vi "Get Ethernet Configuration.vi"(8 "error in (no error)":errorcluster, 11 "Ethernet in":refnum<class "ENET_BS1200.lvclass">) -> (0 "error out":errorcluster, 1 "Configuration Error?":bool, 2 "Ethernet Settings":T1, 3 "Ethernet out":refnum<class "ENET_BS1200.lvclass">)   [LabVIEW 2021, in "BS120x Driver.lvlib" / "ENET_BS1200.lvclass"]
doc: "Retrieve Battery Simulator 1200 Ethernet settings.\n(c) 2019 Bloomy Controls, Inc. All rights reserved."
uses:
  ENET_BS1200.lvclass
  TypeDefs/Ethernet Settings.ctl
  <vilib>/nisyscfg/Close (System).vi
  <vilib>/WebDAVClient/Advanced/Get Buffer.vi
  ENET_BS1200.lvclass/ENET_BS1200.ctl
  <vilib>/WebDAVClient/NI_WebDAV.lvlib
  <resource>/objmgr/nisysapi.rc
  <vilib>/nisyscfg/nisyscfg.lvlib
  BS120x.lvclass
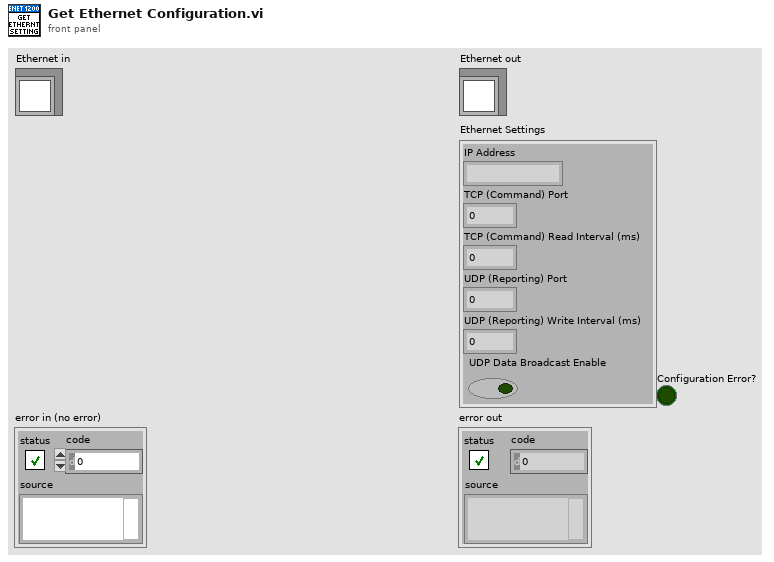
[diagram p1: front panel]
types:
  T1 = typedef "BS120x Driver.lvlib/BS120x.lvclass/Ethernet Settings.ctl" = cluster{"IP Address":string, "TCP (Command) Port":u16, "TCP (Command) Read Interval (ms)":u32, "UDP (Reporting) Port":u16, "UDP (Reporting) Write Interval (ms)":u32, "UDP Data Broadcast Enable":bool}
  T2 = typedef "NI_WebDAV.lvlib/SessionHandle.ctl" = refnum<k1>
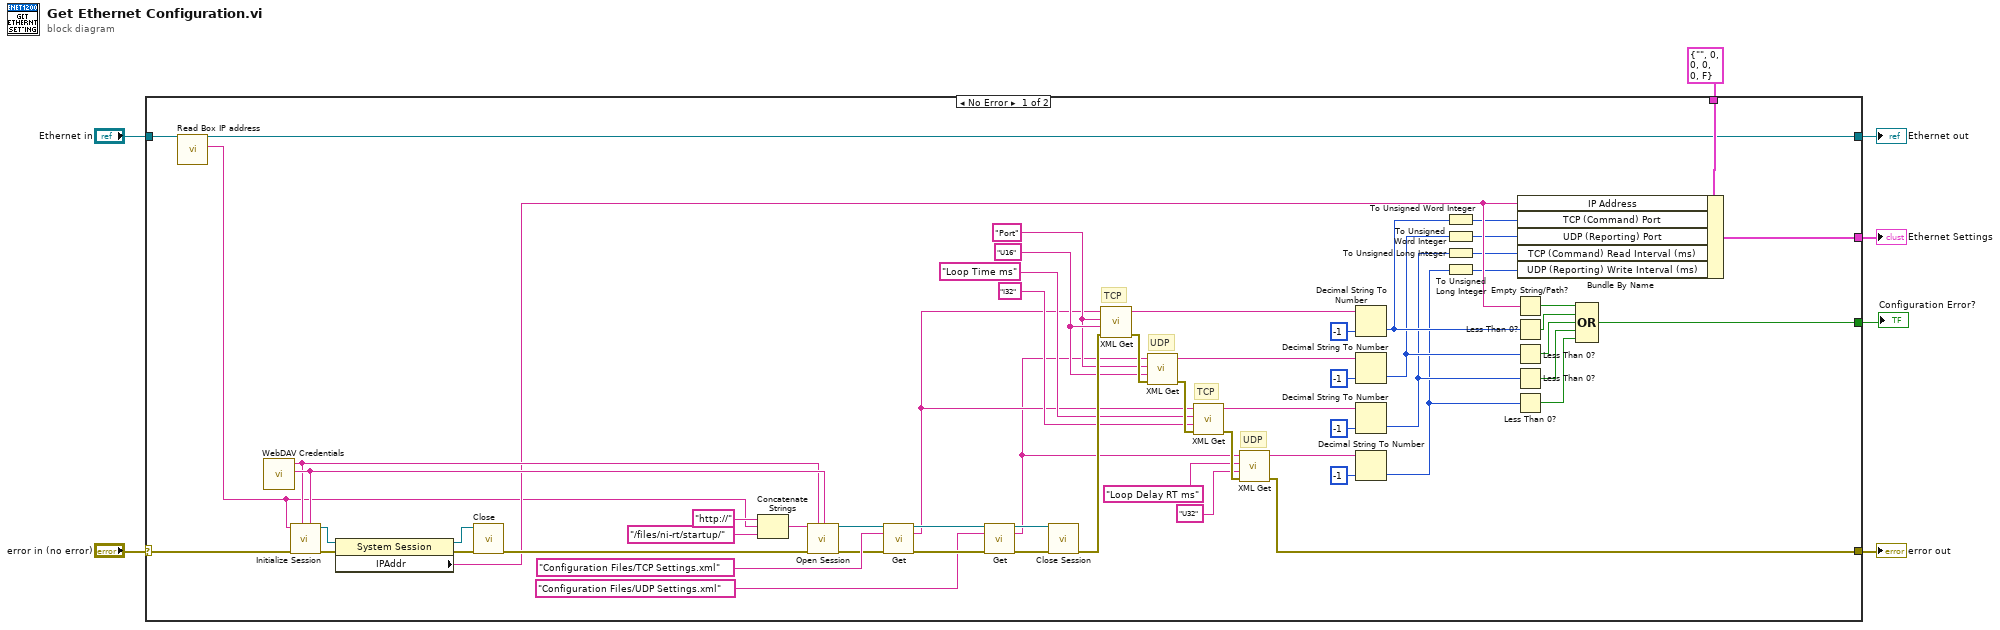
[diagram p0: block diagram]
diagram:
  n1 = case shown="No Error" "error in (no error)" {
    selector: "error in (no error)" -> [w41 w70]
    tunnel: [w46 w70] -> w6
    tunnel: [w9 w69] -> w4
    tunnel: "Ethernet in" -> [w10 w69]
    tunnel: [w66 w68] -> w2
    tunnel: T1 {"IP Address"="", "TCP (Command) Port"=0, "TCP (Command) Read Interval (ms)"=0, "UDP (Reporting) Port"=0, "UDP (Reporting) Write Interval (ms)"=0, "UDP Data Broadcast Enable"=FALSE} ("Ethernet Settings") -> [w67 w68]
    tunnel: [w17 _] -> w1
    frame No Error {
      w43 = "U16" ("Data Type")
      w42 = "Port" ("Parameter")
      # "TCP"
      # "UDP"
      # "UDP"
      # "TCP"
      n2 = call-dynamic "Read Box IP address.vi"("ENET_BS120x in"=w10) -> ("Box IP address"=w8:string, "ENET_BS120x out"=w9:refnum<class "ENET_BS1200.lvclass">)  [unwired: 8 in, 1 out]
      n3 = call "WebDAV Credentials.vi"() -> ("Password"=w35:string, "Username"=w34:string)  [unwired: 10 in]
      n4 = call <vilib>:"Initialize Session.vi"("Password"=w35, "User Name"=w34, "error in (no error)"=w41, "Target (localhost)"=w8) -> ("error out"=w39:errorcluster, "Session out"=w40:refnum<k21>)  [unwired: 6 in]
      n5 = property class="System Session"(reference=w40, error in=w39) -> (reference out=w37:refnum<k21>, error out=w38:errorcluster, "IPAddr"=w27:string)
      n6 = call-poly <vilib>:"Close.vi"("error in (no error)"=w38, "Session in"=w37) -> ("error out"=w36:errorcluster)  [unwired: 9 in]
      n7 = Concatenate Strings("http://" ("string"), w8, "/files/ni-rt/startup/" ("string")) -> (w63:string)
      n8 = call <vilib>:"Open Session.vi"("host uri prefix"=w63, "username"=w34, "password"=w35, "error in (no error)"=w36) -> ("session handle out"=w61:T2, "error out"=w60:errorcluster)  [unwired: 10 in]
      n9 = call-poly <vilib>:"Get.vi"("session handle"=w61, "relative uri"="Configuration Files/TCP Settings.xml" ("string"), "error in (no error)"=w60) -> ("session handle out"=w59:T2, "data"=w12:string, "error out"=w58:errorcluster)  [unwired: 10 in]
      n10 = call-poly <vilib>:"Get.vi"("session handle"=w59, "relative uri"="Configuration Files/UDP Settings.xml" ("string"), "error in (no error)"=w58) -> ("session handle out"=w57:T2, "data"=w11:string, "error out"=w56:errorcluster)  [unwired: 10 in]
      n11 = call <vilib>:"Close Session.vi"("session handle"=w57, "error in (no error)"=w56) -> ("error out"=w53:errorcluster)  [unwired: 13 in]
      n12 = call "XML Get.vi"("error in (no error)"=w53, "Data Type"=w43, "Parameter"=w42, "XML String in"=w12) -> ("error out"=w49:errorcluster, "Value"=w54:string)  [unwired: 6 in]
      n13 = call "XML Get.vi"("error in (no error)"=w49, "Data Type"=w43, "Parameter"=w42, "XML String in"=w11) -> ("error out"=w48:errorcluster, "Value"=w52:string)  [unwired: 6 in]
      n14 = call "XML Get.vi"("error in (no error)"=w48, "Data Type"="I32", "Parameter"="Loop Time ms", "XML String in"=w12) -> ("error out"=w47:errorcluster, "Value"=w51:string)  [unwired: 6 in]
      n15 = call "XML Get.vi"("error in (no error)"=w47, "Data Type"="U32", "Parameter"="Loop Delay RT ms", "XML String in"=w11) -> ("error out"=w46:errorcluster, "Value"=w50:string)  [unwired: 6 in]
      n16 = Decimal String To Number(string=w54, default (0L)=-1 ("default (0 I32)")) -> (number=w26:i32)  [unwired: 1 in, 1 out]
      n17 = Decimal String To Number(string=w52, default (0L)=-1 ("default (0 I32)")) -> (number=w25:i32)  [unwired: 1 in, 1 out]
      n18 = Decimal String To Number(string=w51, default (0L)=-1 ("default (0 I32)")) -> (number=w24:i32)  [unwired: 1 in, 1 out]
      n19 = Decimal String To Number(string=w50, default (0L)=-1 ("default (0 I32)")) -> (number=w23:i32)  [unwired: 1 in, 1 out]
      n20 = To Unsigned Word Integer(number=w26) -> (unsigned 16bit integer=w16:u16)
      n21 = To Unsigned Word Integer(number=w25) -> (unsigned 16bit integer=w15:u16)
      n22 = To Unsigned Long Integer(number=w24) -> (unsigned 32bit integer=w14:u32)
      n23 = To Unsigned Long Integer(number=w23) -> (unsigned 32bit integer=w13:u32)
      n24 = Empty String/Path?(string/path=w27) -> (empty?=w22:bool)
      n25 = Less Than 0?(x=w26) -> (x < 0?=w21:bool)
      n26 = Less Than 0?(x=w25) -> (x < 0?=w20:bool)
      n27 = Less Than 0?(x=w24) -> (x < 0?=w19:bool)
      n28 = Less Than 0?(x=w23) -> (x < 0?=w18:bool)
      n29 = Bundle By Name(cluster=w67, "IP Address"=w27, "TCP (Command) Port"=w16, "UDP (Reporting) Port"=w15, "TCP (Command) Read Interval (ms)"=w14, "UDP (Reporting) Write Interval (ms)"=w13) -> (w66:T1)
      n30 = Compound Arithmetic op=OR(w22, w21, w20, w19, w18) -> (w17:bool)
    }
    frame Error {
    }
  }
  "error out" <- w6
  "Ethernet out" <- w4
  "Ethernet Settings" <- w2
  "Configuration Error?" <- w1
